vi "rethinkdb_json_string_strip.vi"(11 "string in":string) -> (3 "string without first and last":string)   [LabVIEW 2017]
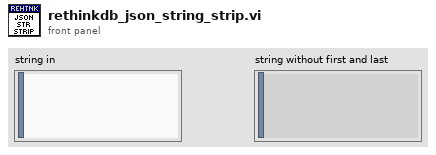
[diagram p1: front panel]
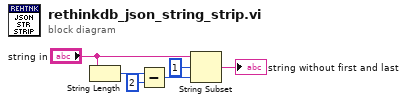
[diagram p0: block diagram]
diagram:
  n1 = String Length(string="string in") -> (length=w3:i32)
  n2 = Subtract(x=w3, y=2) -> (x-y=w1:i32)
  n3 = String Subset(string="string in", offset (0)=1, length (rest)=w1) -> (substring=→"string without first and last":string)
